vi "read large file.vi"() -> ()   [LabVIEW 2016]
uses:
  API/JSON Document Class/json parse/poly instances/json Parse Double - string path.vi
  API/JSON Document Class/json to string/json To Minimized String - string path.vi
  API/JSON Document Class/JSON Document.lvclass
panel:
  out "value":dbl
  out "defaulted?":bool
  out "json string":string
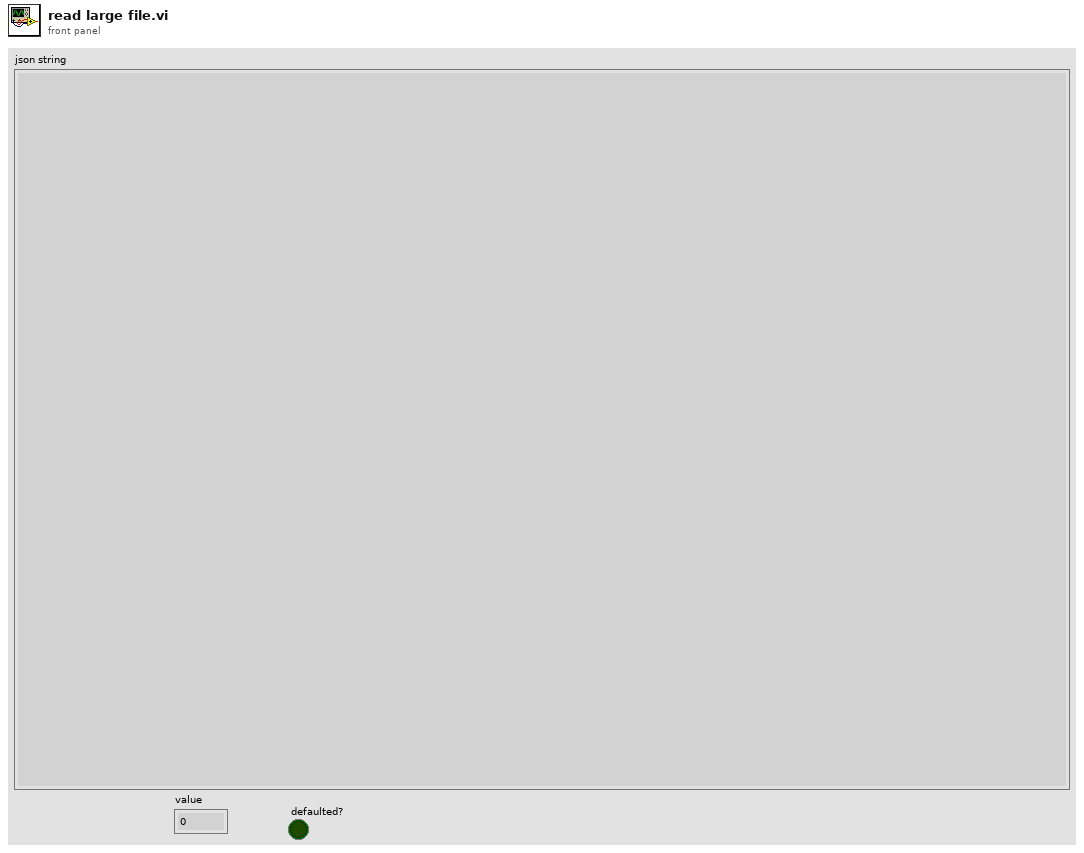
[diagram p1: front panel]
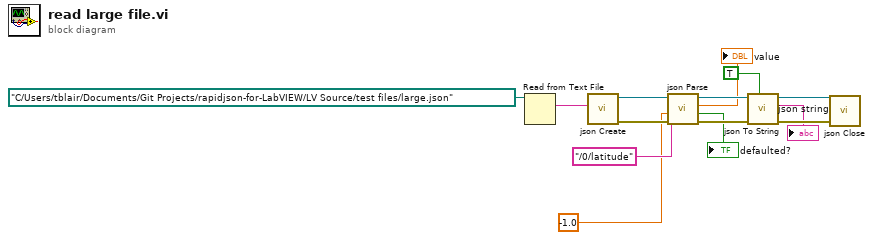
[diagram p0: block diagram]
diagram:
  n1 = Read from Text File(file (use dialog)=path "C:/Users/tblair/Documents/Git Projects/rapidjson-for-LabVIEW/LV Source/test files/large.json") -> (text=w13:string)  [unwired: 3 in, 3 out]
  n2 = call "json Create.vi"("JSON String"=w13) -> ("error out"=w12:errorcluster, "JSON Document out"=w7:refnum<class "JSON Document.lvclass">)  [unwired: 9 in]
  n3 = call-poly "json Parse.vi"("error in (no error)"=w12, "default"=-1.0, "path"="/0/latitude", "JSON Document in"=w7) -> ("error out"=w8:errorcluster, "defaulted?"=→"defaulted?":bool, "value"=→"value":dbl, "JSON Document out"=w6:refnum<class "JSON Document.lvclass">)  [unwired: 4 in]
  n4 = call-poly "json To String.vi"("pretty print?"=TRUE, "error in (no error)"=w8, "JSON Document in"=w6) -> ("error out"=w11:errorcluster, "json string"=→"json string":string, "JSON Document out"=w10:refnum<class "JSON Document.lvclass">)  [unwired: 6 in]
  n5 = call "json Close.vi"("error in (no error)"=w11, "JSON Document in"=w10) -> ()  [unwired: 9 in, 1 out]
